vi "Module Network Stream Decorator.vi"() -> (0 "error out":errorcluster)   [LabVIEW 2025]
uses:
  <extravilib>/ChannelInstances/Event Messenger-c(str,var)/Instantiate.vi
  <extravilib>/ChannelInstances/Event Messenger-c(str,var)/))Channel.vi
  <extravilib>/ChannelInstances/Event Messenger-c(str,var).lvlib
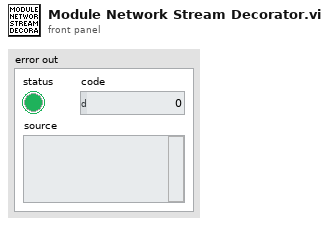
[diagram p1: front panel]
types:
  T1 = typedef "Event Messenger-c(str,var).lvlib/))Channel.ctl" = refnum<queue>
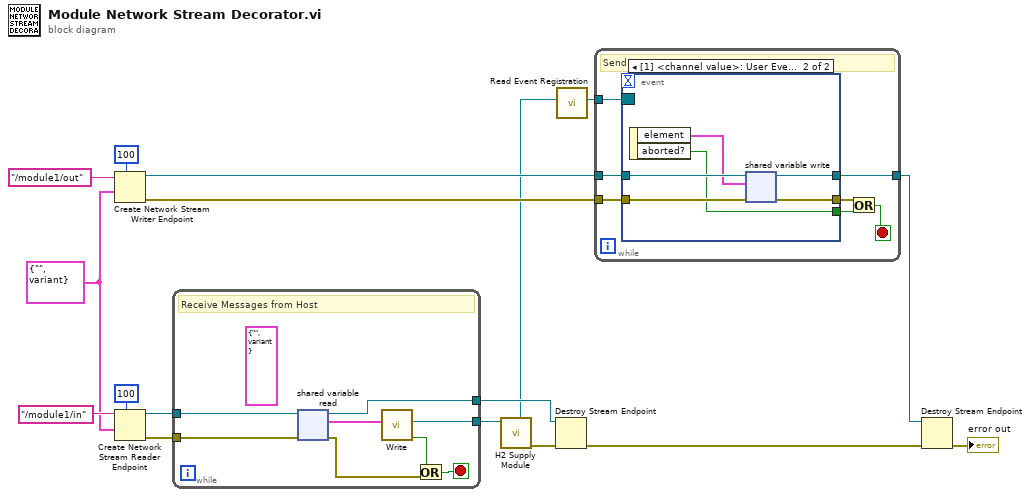
[diagram p0: block diagram]
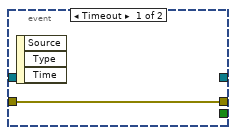
[diagram p2: hidden frame]
diagram:
  w3 = cluster{"cmd":string, "data":variant} {"cmd"="", "data"=variant} ("message")
  n1 = Create Network Stream Writer Endpoint(7:100 ("writer buffer size"), 9:w3, 11:"/module1/out" ("URL")) -> (0:w9:errorcluster, 3:w10:refnum<k21>)  [unwired: 4 in]
  n2 = Create Network Stream Reader Endpoint(7:100 ("reader buffer size"), 9:w3, 11:"/module1/in" ("URL")) -> (0:w17:errorcluster, 3:w16:refnum<k21>)  [unwired: 4 in]
  n3 = while {
    tunnel: w17 -> [w19]
    tunnel: w16 -> [w18]
    tunnel: [w25] -> w13
    tunnel: [w24] -> w12
    stop <- w21 stop-if-true
    (unwired) cluster{"cmd":string, "data":variant} {"cmd"="", "data"=variant} ("message")
    # "Receive Messages from Host"
    n4 = shared-variable-read(w18, w19) -> (w25:refnum<k21>, w22:errorcluster, w23:cluster{"cmd":string, "data":variant})  [unwired: 1 in, 1 out]
    n5 = call <extravilib>:"Write.vi"("element"=w23) -> ("done?"=w20:bool, "channel"=w24:T1)  [unwired: 9 in]
    n6 = Or(x=w20, y=w22) -> (x .or. y?=w21:bool)
  }
  n7 = call "H2 Supply Module.vi"("Message Input"=w12) -> ("error out"=w14:errorcluster, "Message Output"=w8:T1)  [unwired: 9 in]
  n8 = Destroy Stream Endpoint(8:w14, 11:w13) -> (0:w7:errorcluster)
  n9 = call <extravilib>:"Read Event Registration.vi"("channel"=w8) -> ("event registration refnum"=w5:refnum<event-registration>)  [unwired: 10 in]
  n10 = while {
    tunnel: w9 -> [w30]
    tunnel: w10 -> [w31]
    tunnel: w5 -> [w32]
    tunnel: [w29] -> w4
    stop <- w27 stop-if-true
    # "Send Messages to Host"
    n11 = event shown="[1] <channel value>: User Event" {
      selector: w32 -> [_ _]
      dyn-events: _ -> [_ _]
      timeout: _ -> [_ _]
      tunnel: w31 -> [_ w38]
      tunnel: w30 -> [w33 w39]
      tunnel: [_ w36] -> w29
      tunnel: [w33 w35] -> w28
      tunnel: [_ w34] -> w26
      event Timeout {
        n12 = event-data() -> ()  [unwired: 1 in, 3 out]
      }
      event User Event {
        n13 = event-data() -> ("element"=w37:cluster{"cmd":string, "data":variant}, "aborted?"=w34:bool)  [unwired: 1 in]
        n14 = shared-variable-write(w38, w39, w37) -> (w36:refnum<k21>, w35:errorcluster)  [unwired: 1 in, 1 out]
      }
    }
    n15 = Or(x=w28, y=w26) -> (x .or. y?=w27:bool)
  }
  n16 = Destroy Stream Endpoint(8:w7, 11:w4) -> (0:→"error out":errorcluster)
